vi "ALR scada.vi"(8 "error in (no error)":errorcluster, 10 "OPC UA client refnum in":T1, 11 "ALR_State in":T2) -> (0 "error out":errorcluster, 3 "ALR_State out":T2)   [LabVIEW 2019, in "Alarms.lvlib"]
uses:
  Alarms.lvlib
  Ctl/ALRs_State.ctl
  <vilib>/OPCUA/controls/OPC UA Client Refnum.ctl
  <vilib>/OPCUA/controls/NodeIds.ctl
  <vilib>/OPCUA/controls/NodeId.ctl
  <vilib>/OPCUA/client/Multiple Read Bool Array.vi
  <vilib>/OPCUA/client/Multiple Read UInt32 Array.vi
  <vilib>/OPCUA/NI OPC UA Client.lvlib
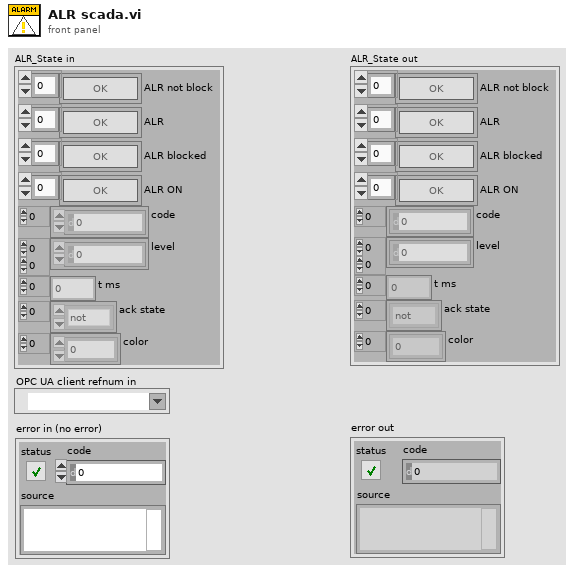
[diagram p1: front panel]
types:
  T1 = typedef "OPC UA Client Refnum.ctl" = refnum<k21>
  T2 = typedef "Alarms.lvlib/ALRs_State.ctl" = cluster{"ALR not block":bool[], "ALR":bool[], "ALR blocked":bool[], "ALR ON":bool[], "code":i32[], "level":i32[][], "t ms":u32[], "ack state":enum32{"not", "tripped", "reset", "ack"}[], "color":u32[]}
  T3 = typedef "NodeIds.ctl" = T4[]
  T4 = typedef "NodeId.ctl" = string
  T5 = typedef "OPC UA StatusCode.ctl" = u32
  T6 = cluster{"node ID":T4, "values ":bool[], "timestamp":timestamp, "status":T5}[]
  T7 = cluster{"node ID":T4, "values ":bool[], "timestamp":timestamp, "status":T5}
  T8 = cluster{"node ID":T4, "values ":u32[], "timestamp":timestamp, "status":T5}[]
  T9 = cluster{"node ID":T4, "values ":u32[], "timestamp":timestamp, "status":T5}
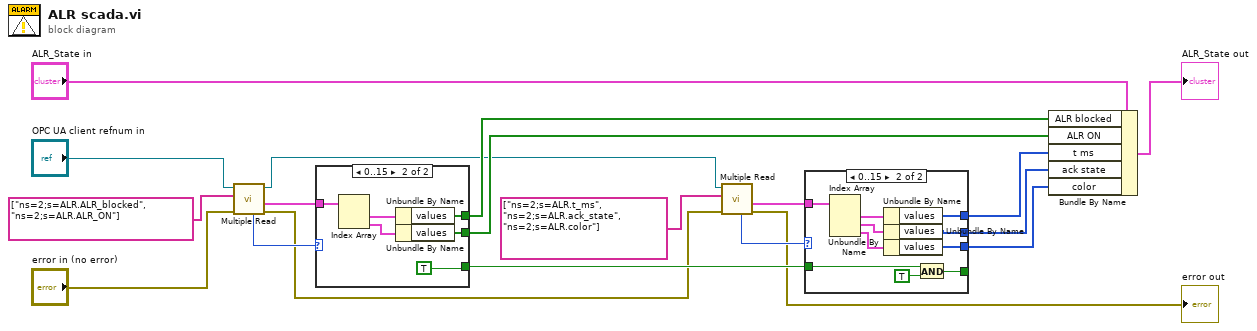
[diagram p0: block diagram]
diagram:
  n1 = call-poly <vilib>:"Multiple Read.vi"("error in (no error)"="error in (no error)", "node IDs"=T3 ["ns=2;s=ALR.ALR_blocked", "ns=2;s=ALR.ALR_ON"] ("OPC UA.node IDs"), "OPC UA client refnum in"="OPC UA client refnum in") -> ("error out"=w2:errorcluster, "results"=w15:T6, "OPC UA client refnum out"=w4:T1, "service status"=w16:T5)  [unwired: 5 in]
  n2 = case shown="0..15" w16 {
    tunnel: w15 -> [_ w24]
    tunnel: [_ TRUE] -> w10
    tunnel: [_ w22] -> w6
    tunnel: [_ w20] -> w5
    frame 16.., Default {
    }
    frame 0..15 {
      n3 = Index Array(array=w24) -> (element #1=w25:T7, element #2=w21:T7)  [unwired: 2 in]
      n4 = Unbundle By Name(w25) -> ("values"=w22:bool[])
      n5 = Unbundle By Name(w21) -> ("values"=w20:bool[])
    }
  }
  n6 = call-poly <vilib>:"Multiple Read.vi"("error in (no error)"=w2, "node IDs"=T3 ["ns=2;s=ALR.t_ms", "ns=2;s=ALR.ack_state", "ns=2;s=ALR.color"] ("OPC UA.node IDs"), "OPC UA client refnum in"=w4) -> ("error out"=→"error out":errorcluster, "results"=w12:T8, "service status"=w11:T5)  [unwired: 5 in, 1 out]
  n7 = case shown="0..15" w11 {
    tunnel: w12 -> [_ w34]
    tunnel: [_ w33] -> w9
    tunnel: w10 -> [_ w32]
    tunnel: [_ w30] -> _
    tunnel: [_ w28] -> w8
    tunnel: [_ w26] -> w7
    frame 16.., Default {
    }
    frame 0..15 {
      n8 = Index Array(array=w34) -> (element #1=w35:T9, element #2=w29:T9, element #3=w27:T9)  [unwired: 3 in]
      n9 = Unbundle By Name(w35) -> ("values"=w33:u32[])
      n10 = Unbundle By Name(w29) -> ("values"=w28:u32[])
      n11 = Unbundle By Name(w27) -> ("values"=w26:u32[])
      n12 = And(x=w32, y=TRUE) -> (x .and. y?=w30:bool)
    }
  }
  n13 = Bundle By Name(cluster="ALR_State in", "ALR blocked"=w6, "ALR ON"=w5, "t ms"=w9, "ack state"=w8, "color"=w7) -> (→"ALR_State out":T2)
